vi "3d_display2.vi"() -> ()   [LabVIEW 2009]
doc: "This example demonstrates some fundamental concepts for the 3D picture control. Concepts covered include:\n\n-Object creation\n-Texturing\n-Object movement\n-Object hierarchy"
uses:
  <vilib>/Utility/miscctls.llb/LVRectTypeDef.ctl
  <vilib>/picture/3D Picture Control/NI_3D Picture Control.lvlib
  <vilib>/Analysis/NI_AALBase.lvlib
panel:
  out "Numeric 2":dbl
  out "Numeric":dbl
  in  "Set Start Time (s)":dbl
  in  "X":dbl
  in  "Z":dbl
  in  "Calibrate Z":bool
  in  "Calibrate Y":bool
  in  "Calibrate X":bool
  out "angle 2":dbl
  out "angle 1":dbl
  out "X mean acceleration":dbl format="%0.4f"
  out "Y mean acceleration":dbl format="%0.4f"
  out "X mean volts":dbl format="%0.4f"
  out "Y mean volts":dbl format="%0.4f"
  out "Z mean acceleration":dbl format="%0.4f"
  out "Z mean volts":dbl format="%0.4f"
  in  "z gain":dbl=5.0
  in  "z offset":dbl=1.25
  in  "y gain":dbl=5.0
  in  "y offset":dbl=1.25
  in  "x gain":dbl=5.0
  in  "x offset":dbl=1.25
  in  "Render Dest":enum16{"Scene Window", "Scene Display"}(ring)
  in  "Camera Controller":enum16{"None", "Spherical", "Flying"}(ring)=enum."Spherical"
  out "Scene Display":refnum<vi>(3d-picture)
  in  "stop":bool
  # "Select 'Render Dest'\nbefore running!"
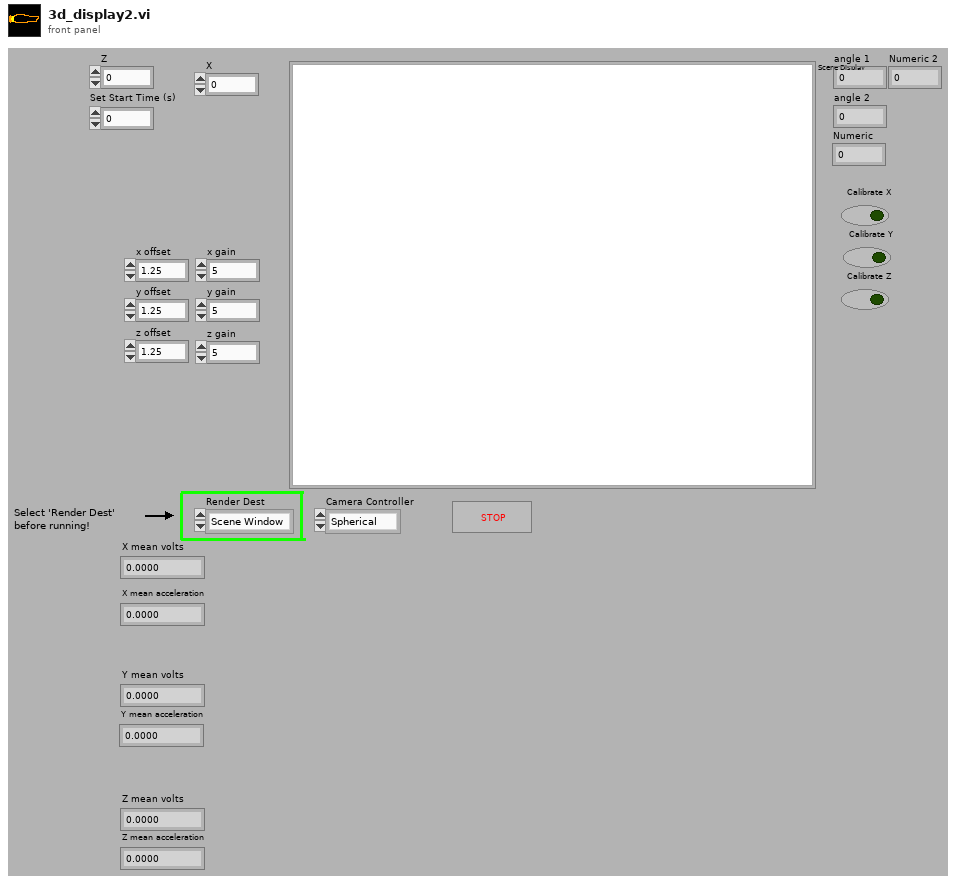
[diagram p1: front panel]
types:
  T1 = typedef "LVRectTypeDef.ctl" = cluster{"Left":i16, "Top":i16, "Right":i16, "Bottom":i16}
  T2 = enum16{"Open", "Minimized", "Maximized", "Hidden"}
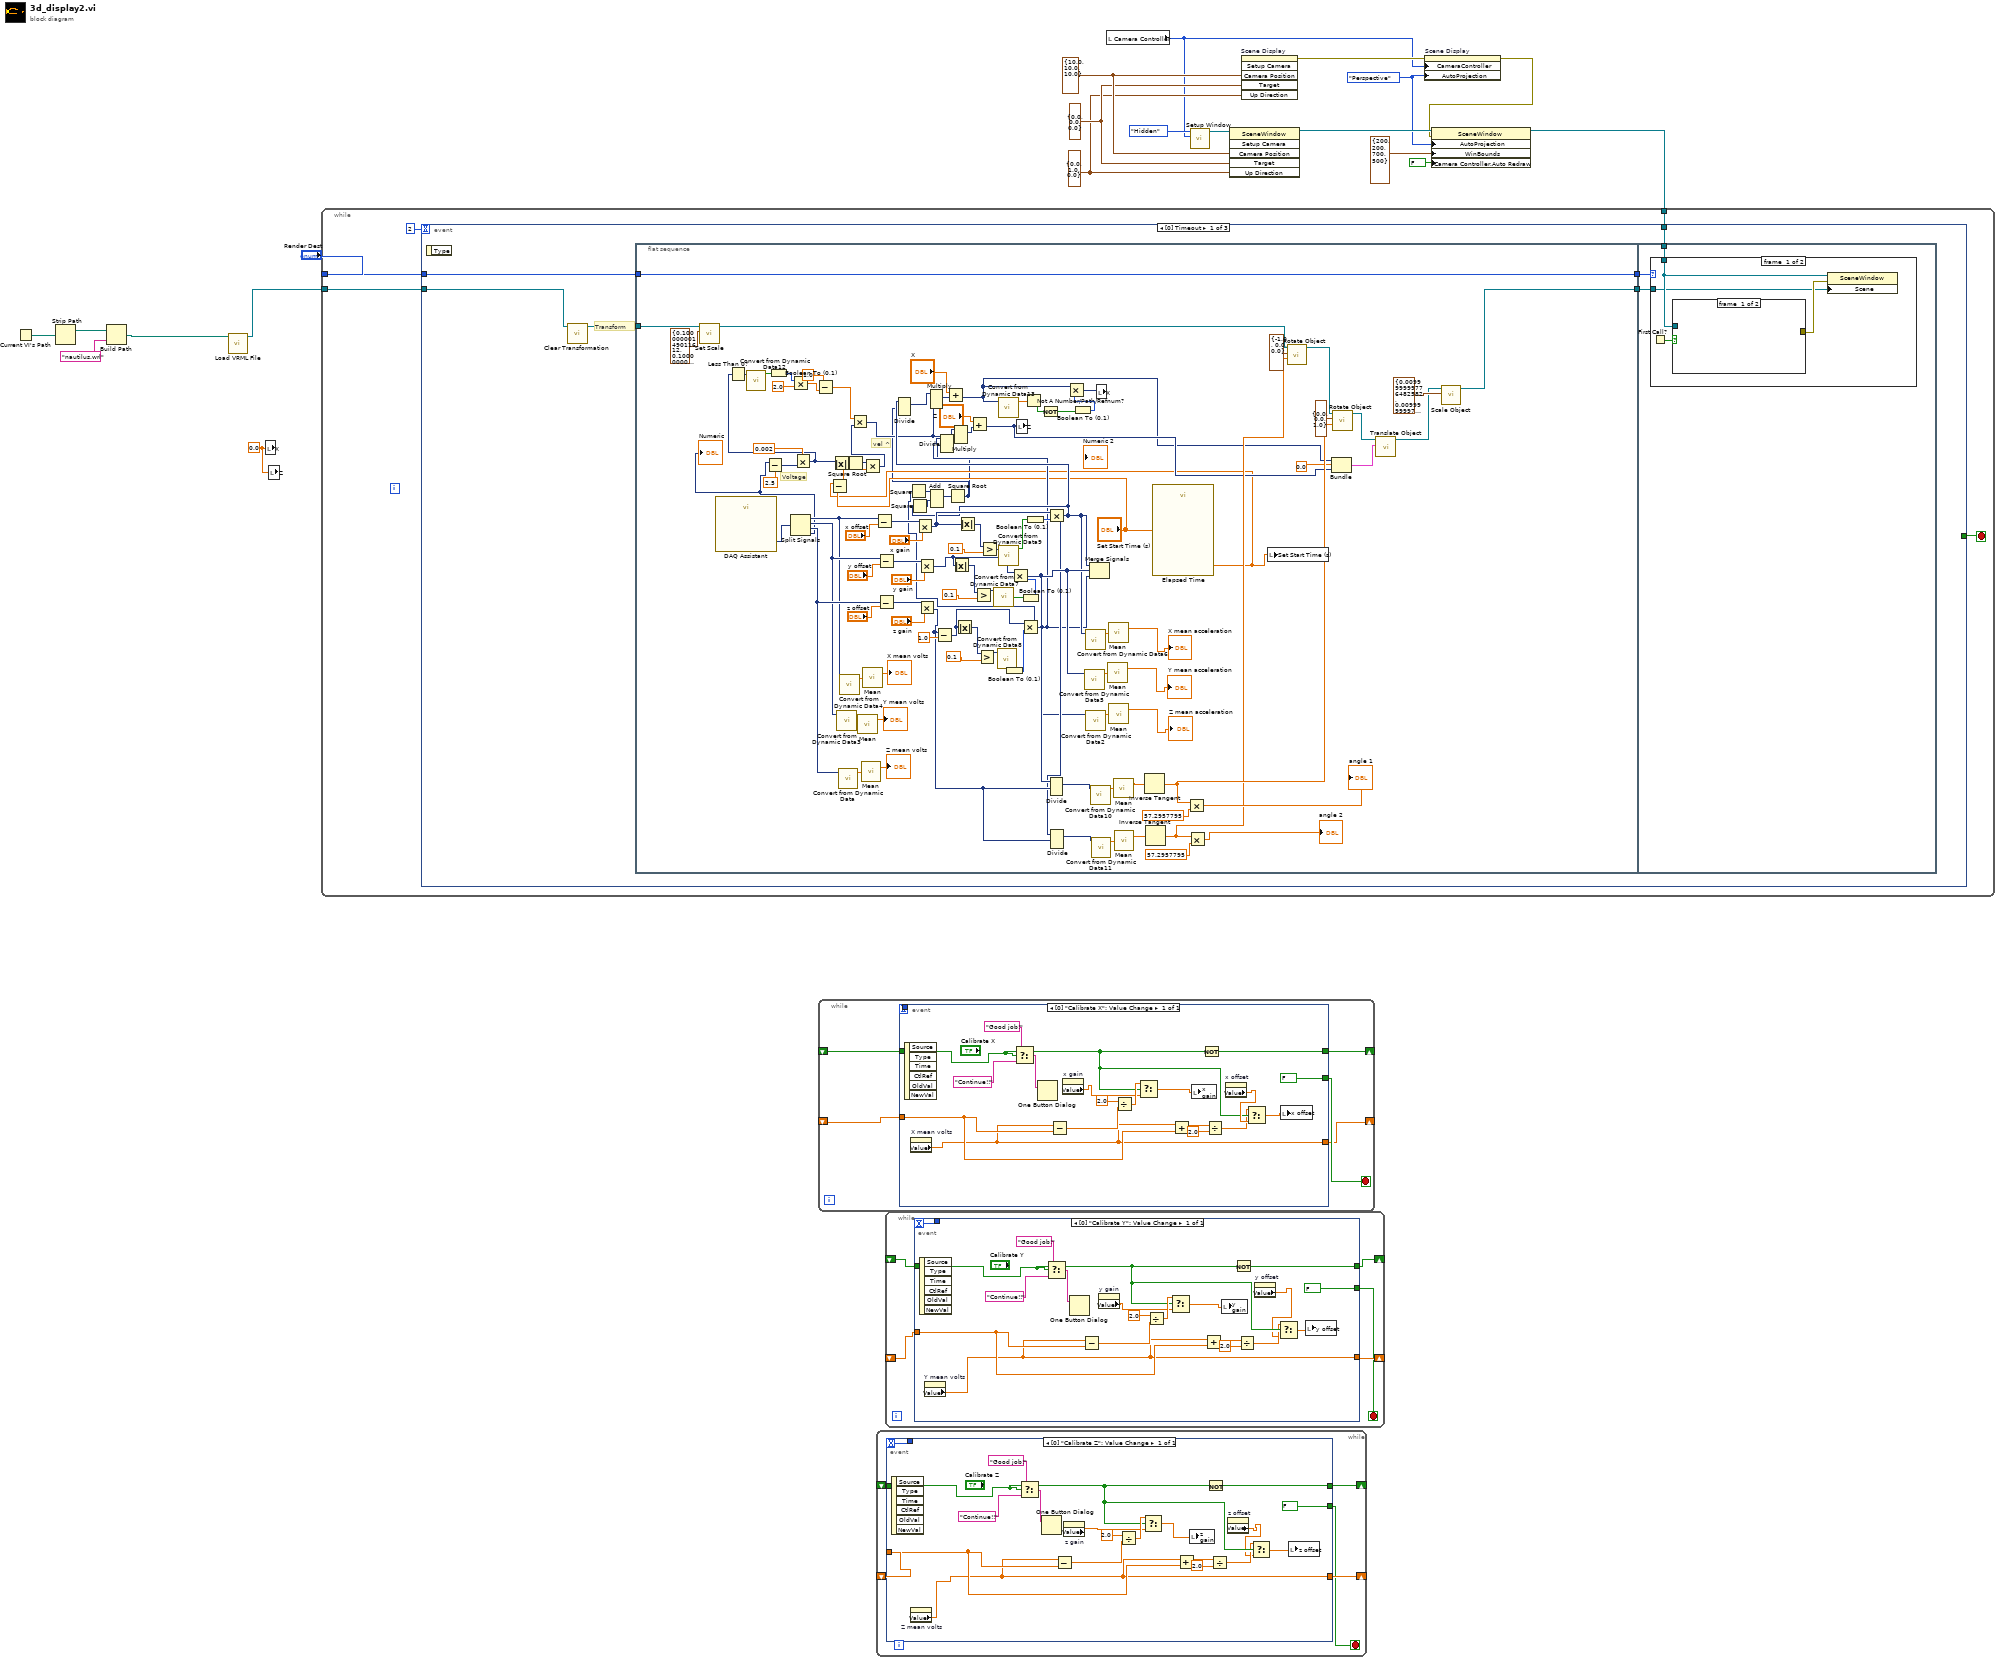
[diagram p0: block diagram]
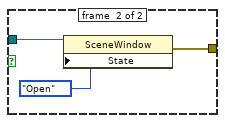
[diagram p2: hidden frame]
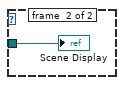
[diagram p3: hidden frame]
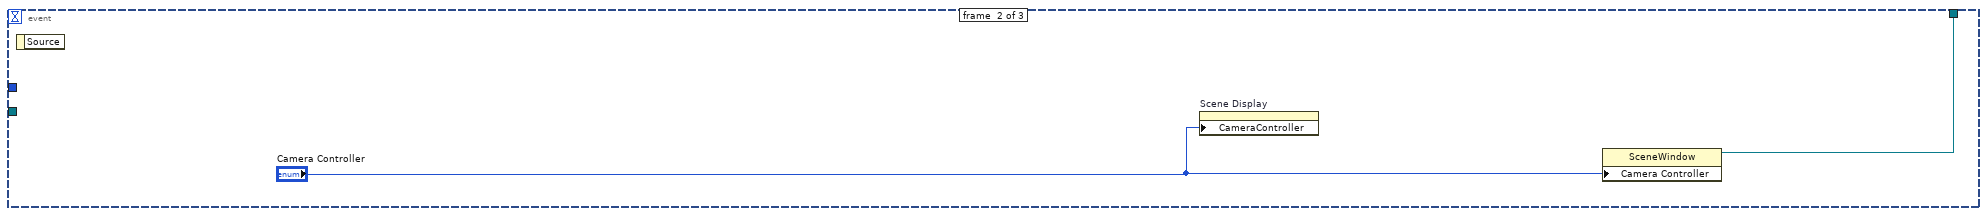
[diagram p4: hidden frame]
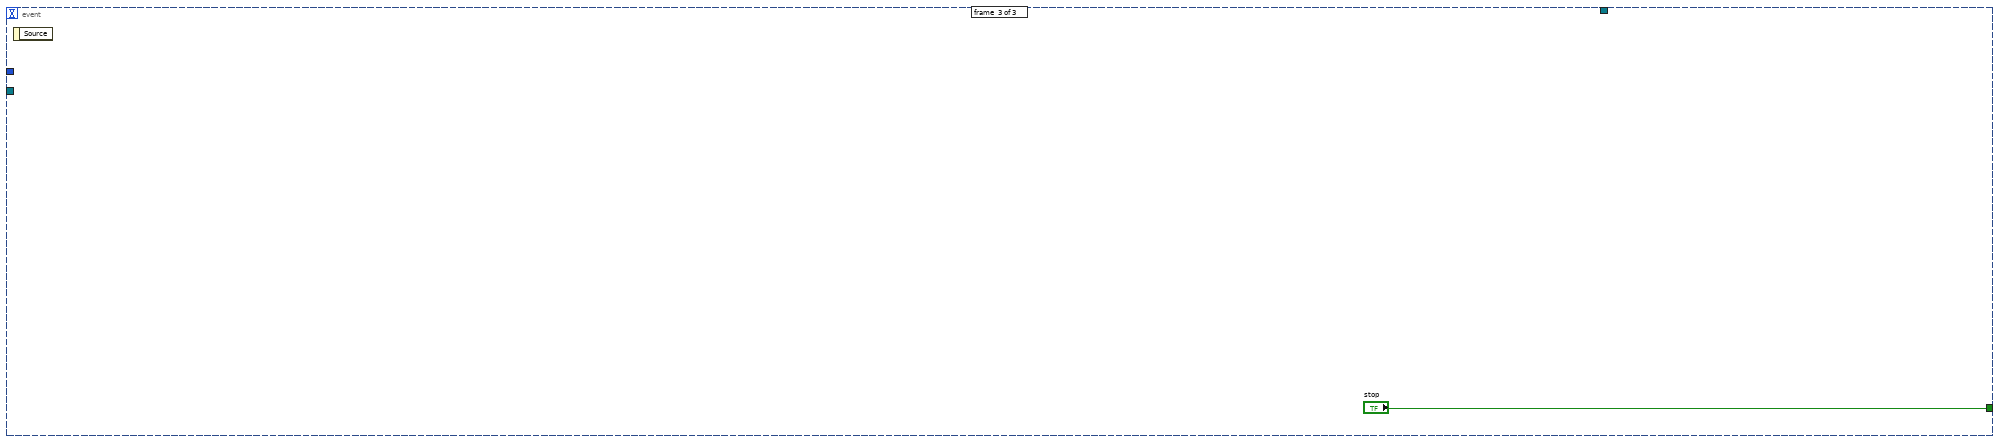
[diagram p5: hidden frame]
diagram:
  w1 = 0.0 ("X")
  w13 = enum16{"None", "Perspective", "Orthographic"}."Perspective" ("Auto Projection Mode")
  w16 = cluster{"X":sgl, "Y":sgl, "Z":sgl} {"X"=0.0, "Y"=1.0, "Z"=0.0} ("Up Direction")
  w17 = cluster{"X":sgl, "Y":sgl, "Z":sgl} {"X"=0.0, "Y"=0.0, "Z"=0.0} ("Target")
  w18 = cluster{"X":sgl, "Y":sgl, "Z":sgl} {"X"=10.0, "Y"=10.0, "Z"=10.0} ("Camera Position")
  n1 = Current VI's Path() -> (path=w5:path)
  n2 = Strip Path(path=w5) -> (stripped path=w6:path)  [unwired: 1 out]
  n3 = Build Path(base path=w6, name or relative path="nautilus.wrl") -> (appended path=w3:path)
  n4 = call <vilib>:"Load VRML File.vi"("Path"=w3) -> ("Scene:Read Scene File"=w2:refnum<vi>)  [unwired: 9 in, 1 out]
  n5 = local write "X"(w1) -> ()
  n6 = local write "Z"(w1) -> ()
  n7 = while {
    shift-right: [w23] -> _
    shift-left: _ -> [w24]
    shift-right: [w22] -> _
    shift-left: _ -> [w21]
    stop <- w25 stop-if-true
    n8 = event shown="[0] \"Calibrate X\": Value Change" {
      selector: _ -> [_]
      dyn-events: _ -> [_]
      timeout: _ -> [w44]
      tunnel: [w44] -> _
      tunnel: [FALSE ("Run")] -> w25
      tunnel: w24 -> [w31]
      tunnel: [w39] -> w23
      tunnel: [w26] -> w22
      tunnel: w21 -> [w30]
      event [0] "Calibrate X": Value Change {
        n9 = event-data() -> ()  [unwired: 1 in, 6 out]
        n10 = property on="X mean volts" class="DigNum (strict)"() -> ("Value"=w26:dbl)  [unwired: 2 in, 2 out]
        n11 = Select(t="Good job!" ("message"), s=w31, f="Continue!!" ("message")) -> (s? t:f=w43:string)
        n12 = One Button Dialog(message=w43) -> ()  [unwired: 1 in, 1 out]
        n13 = Subtract(x=w26, y=w30) -> (x-y=w37:dbl)
        n14 = property on="x gain" class="DigNum (strict)"() -> ("Value"=w35:dbl)  [unwired: 2 in, 2 out]
        n15 = Divide(x=2.0, y=w37) -> (x/y=w36:dbl)
        n16 = Select(t=w36, s=w31, f=w35) -> (s? t:f=w34:dbl)
        n17 = Add(x=w26, y=w30) -> (x+y=w28:dbl)
        n18 = local write "x gain"(w34) -> ()
        n19 = Not(x=w31) -> (.not. x?=w39:bool)
        n20 = Divide(x=w28, y=2.0) -> (x/y=w27:dbl)
        n21 = property on="x offset" class="DigNum (strict)"() -> ("Value"=w32:dbl)  [unwired: 2 in, 2 out]
        n22 = Select(t=w27, s=w31, f=w32) -> (s? t:f=w33:dbl)
        n23 = local write "x offset"(w33) -> ()
      }
    }
  }
  n24 = while {
    shift-right: [w47] -> _
    shift-left: _ -> [w46]
    shift-right: [w49] -> _
    shift-left: _ -> [w48]
    stop <- w45 stop-if-true
    n25 = event shown="[0] \"Calibrate Z\": Value Change" {
      selector: _ -> [_]
      dyn-events: _ -> [_]
      timeout: _ -> [w68]
      tunnel: [w68] -> _
      tunnel: w48 -> [w60]
      tunnel: [w64] -> w49
      tunnel: [w50] -> w47
      tunnel: w46 -> [w59]
      tunnel: [FALSE ("Run")] -> w45
      event [0] "Calibrate Z": Value Change {
        n26 = event-data() -> ()  [unwired: 1 in, 6 out]
        n27 = property on="Z mean volts" class="DigNum (strict)"() -> ("Value"=w50:dbl)  [unwired: 2 in, 2 out]
        n28 = Select(t="Good job!" ("message"), s=w60, f="Continue!!" ("message")) -> (s? t:f=w67:string)
        n29 = One Button Dialog(message=w67) -> ()  [unwired: 1 in, 1 out]
        n30 = Subtract(x=w50, y=w59) -> (x-y=w62:dbl)
        n31 = property on="z gain" class="DigNum (strict)"() -> ("Value"=w54:dbl)  [unwired: 2 in, 2 out]
        n32 = Divide(x=2.0, y=w62) -> (x/y=w61:dbl)
        n33 = Select(t=w61, s=w60, f=w54) -> (s? t:f=w52:dbl)
        n34 = Add(x=w50, y=w59) -> (x+y=w57:dbl)
        n35 = local write "z gain"(w52) -> ()
        n36 = Not(x=w60) -> (.not. x?=w64:bool)
        n37 = Divide(x=w57, y=2.0) -> (x/y=w56:dbl)
        n38 = property on="z offset" class="DigNum (strict)"() -> ("Value"=w53:dbl)  [unwired: 2 in, 2 out]
        n39 = Select(t=w56, s=w60, f=w53) -> (s? t:f=w55:dbl)
        n40 = local write "z offset"(w55) -> ()
      }
    }
  }
  n41 = while {
    shift-right: [w73] -> _
    shift-left: _ -> [w72]
    shift-right: [w70] -> _
    shift-left: _ -> [w71]
    stop <- w69 stop-if-true
    n42 = event shown="[0] \"Calibrate Y\": Value Change" {
      selector: _ -> [_]
      dyn-events: _ -> [_]
      timeout: _ -> [w92]
      tunnel: [w92] -> _
      tunnel: w72 -> [w84]
      tunnel: [w88] -> w73
      tunnel: [w74] -> w70
      tunnel: w71 -> [w83]
      tunnel: [FALSE ("Run")] -> w69
      event [0] "Calibrate Y": Value Change {
        n43 = event-data() -> ()  [unwired: 1 in, 6 out]
        n44 = property on="Y mean volts" class="DigNum (strict)"() -> ("Value"=w74:dbl)  [unwired: 2 in, 2 out]
        n45 = Select(t="Good job!" ("message"), s=w84, f="Continue!!" ("message")) -> (s? t:f=w91:string)
        n46 = One Button Dialog(message=w91) -> ()  [unwired: 1 in, 1 out]
        n47 = Subtract(x=w74, y=w83) -> (x-y=w86:dbl)
        n48 = property on="y gain" class="DigNum (strict)"() -> ("Value"=w79:dbl)  [unwired: 2 in, 2 out]
        n49 = Divide(x=2.0, y=w86) -> (x/y=w85:dbl)
        n50 = Select(t=w85, s=w84, f=w79) -> (s? t:f=w78:dbl)
        n51 = Add(x=w74, y=w83) -> (x+y=w81:dbl)
        n52 = local write "y gain"(w78) -> ()
        n53 = Not(x=w84) -> (.not. x?=w88:bool)
        n54 = Divide(x=w81, y=2.0) -> (x/y=w80:dbl)
        n55 = property on="y offset" class="DigNum (strict)"() -> ("Value"=w77:dbl)  [unwired: 2 in, 2 out]
        n56 = Select(t=w80, s=w84, f=w77) -> (s? t:f=w76:dbl)
        n57 = local write "y offset"(w76) -> ()
      }
    }
  }
  n58 = local read "Camera Controller"() -> (w10:enum16{"None", "Spherical", "Flying"})
  n59 = call <vilib>:"Setup Window.vi"("Camera Controller"=w10, "Window State"=T2."Hidden") -> ("New Window Refnum"=w12:refnum<vi>)  [unwired: 1 in, 8 out]
  n60 = invoke class="SceneWindow" method="Setup Camera"(reference=w12, "Camera Position"=w18, "Target"=w17, "Up Direction"=w16) -> (reference out=w20:refnum<vi>)  [unwired: 2 in, 5 out]
  n61 = invoke on="Scene Display" class="SceneGraphDisp (strict)" method="Setup Camera"("Camera Position"=w18, "Target"=w17, "Up Direction"=w16) -> (error out=w15:errorcluster)  [unwired: 3 in, 5 out]
  n62 = property on="Scene Display" class="SceneGraphDisp (strict)"(error in=w15, "CameraController"=w10, "AutoProjection"=w13) -> (error out=w14:errorcluster)  [unwired: 1 in, 1 out]
  n63 = property class="SceneWindow"(reference=w20, error in=w14, "AutoProjection"=w13, "WinBounds"=T1 {"Left"=200, "Top"=200, "Right"=700, "Bottom"=500} ("Window Bounds"), "Camera Controller.Auto Redraw"=FALSE ("Camera Controller:Auto Redraw")) -> (reference out=w8:refnum<vi>)  [unwired: 1 out]
  n64 = while {
    tunnel: w8 -> [w97]
    tunnel: w2 -> [w96]
    tunnel: "Render Dest" -> [w93]
    stop <- w94 stop-if-true
    n65 = event shown="[0] Timeout" {
      selector: _ -> [_ _ _]
      dyn-events: _ -> [_ _ _]
      timeout: 2 -> [_ _ _]
      tunnel: w97 -> [w103 w225 _]
      tunnel: w96 -> [w99 _ _]
      tunnel: [_ _ "stop"] -> w94
      tunnel: w93 -> [w100 _ _]
      event #0 {
        # "Transform"
        n66 = event-data() -> ()  [unwired: 2 out]
        n67 = call <vilib>:"Clear Transformation.vi"("Object Refnum In"=w99) -> ("Object Refnum Out"=w102:refnum<vi>)  [unwired: 1 in, 9 out]
        n68 = flat-sequence {
          tunnel: w102 -> [w113]
          tunnel: [w212] -> w101
          tunnel: w100 -> [w212]
          tunnel: [w209] -> w98
          tunnel: w103 -> [w215]
          tunnel: w101 -> [w214]
          tunnel: w98 -> [w213]
          frame #0 {
            # "vel ^"
            # "Voltage"
            n69 = call <vilib>:"Set Scale.vi"("Scale"=cluster{"X":sgl, "Y":sgl, "Z":sgl} {"X"=0.1, "Y"=0.1, "Z"=0.1}, "Scene Object"=w113) -> ("Scaled Object"=w112:refnum<vi>)  [unwired: 8 in, 1 out]
            n70 = call "DAQ Assistant"() -> ("data"=w152:dynamicdata)  [unwired: 17 in, 2 out]
            n71 = Split Signals(w152) -> (w192:dynamicdata, w194:dynamicdata, w197:dynamicdata, w118:dynamicdata)  [unwired: 4 in]
            "Numeric" <- w118
            n72 = Subtract(x=w118, y=2.5) -> (x-y=w147:dynamicdata)
            n73 = Multiply(x=0.002, y=w147) -> (x*y=w117:dynamicdata)
            n74 = Less Than 0?(x=w117) -> (x < 0?=w126:dynamicdata)
            n75 = call "Convert from Dynamic Data12"("Dynamic Data Type"=w126) -> ("Scalar"=w125:bool)  [unwired: 3 in]
            n76 = Boolean To (0,1)(Boolean=w125) -> (0, 1=w123:i16)
            n77 = Multiply(x=w123, y=2.0) -> (x*y=w121:dbl)
            n78 = Subtract(x=1.0 ("y"), y=w121) -> (x-y=w116:dbl)
            n79 = Absolute Value(x=w117) -> (abs(x)=w120:dynamicdata)
            n80 = call "Convert from Dynamic Data3"("Dynamic Data Type"=w194) -> ("Array"=w193:dbl[])  [unwired: 3 in]
            n81 = call "Convert from Dynamic Data"("Dynamic Data Type"=w197) -> ("Array"=w199:dbl[])  [unwired: 3 in]
            n82 = call "Convert from Dynamic Data4"("Dynamic Data Type"=w192) -> ("Array"=w191:dbl[])  [unwired: 3 in]
            n83 = Square Root(x=w120) -> (sqrt(x)=w119:dynamicdata)
            n84 = call <vilib>:"Mean.vi"("X"=w193) -> ("mean"=→"Y mean volts":dbl)  [unwired: 1 out]
            n85 = call <vilib>:"Mean.vi"("X"=w199) -> ("mean"=→"Z mean volts":dbl)  [unwired: 1 out]
            n86 = call <vilib>:"Mean.vi"("X"=w191) -> ("mean"=→"X mean volts":dbl)  [unwired: 1 out]
            n87 = Subtract(x=w192, y="x offset") -> (x-y=w208:dynamicdata)
            n88 = Subtract(x=w194, y="y offset") -> (x-y=w204:dynamicdata)
            n89 = Subtract(x=w197, y="z offset") -> (x-y=w186:dynamicdata)
            n90 = Multiply(x=w208, y="x gain") -> (x*y=w167:dynamicdata)
            n91 = Multiply(x=w204, y="y gain") -> (x*y=w185:dynamicdata)
            n92 = Multiply(x=w186, y="z gain") -> (x*y=w156:dynamicdata)
            n93 = Subtract(x=w156, y=1.0) -> (x-y=w173:dynamicdata)
            n94 = Absolute Value(x=w185) -> (abs(x)=w184:dynamicdata)
            n95 = Absolute Value(x=w173) -> (abs(x)=w179:dynamicdata)
            n96 = Absolute Value(x=w167) -> (abs(x)=w172:dynamicdata)
            n97 = Greater?(x=w184, y=0.1) -> (0:w181:dynamicdata)
            n98 = Greater?(x=w179, y=0.1) -> (0:w177:dynamicdata)
            n99 = Greater?(x=w172, y=0.1) -> (0:w169:dynamicdata)
            n100 = call "Convert from Dynamic Data7"("Dynamic Data Type"=w181) -> ("Scalar"=w180:bool)  [unwired: 3 in]
            n101 = call "Convert from Dynamic Data8"("Dynamic Data Type"=w177) -> ("Scalar"=w176:bool)  [unwired: 3 in]
            n102 = call "Convert from Dynamic Data9"("Dynamic Data Type"=w169) -> ("Scalar"=w168:bool)  [unwired: 3 in]
            n103 = Boolean To (0,1)(Boolean=w176) -> (0, 1=w175:i16)
            n104 = Boolean To (0,1)(Boolean=w180) -> (0, 1=w182:i16)
            n105 = Multiply(x=w185, y=w182) -> (x*y=w162:dynamicdata)
            n106 = Multiply(x=w173, y=w175) -> (x*y=w136:dynamicdata)
            n107 = Square(x=w136) -> (x^2=w142:dynamicdata)
            n108 = Boolean To (0,1)(Boolean=w168) -> (0, 1=w170:i16)
            n109 = Divide(1:w156, 2:w162) -> (0:w164:dynamicdata)  [unwired: 1 in, 1 out]
            n110 = Multiply(x=w167, y=w170) -> (x*y=w137:dynamicdata)
            n111 = Square(x=w137) -> (x^2=w143:dynamicdata)
            n112 = Add(1:w143, 2:w142) -> (0:w141:dynamicdata)  [unwired: 1 in, 1 out]
            n113 = Square Root(x=w141) -> (sqrt(x)=w110:dynamicdata)
            n114 = Divide(1:w110, 2:w137) -> (0:w139:dynamicdata)  [unwired: 1 in, 1 out]
            n115 = Divide(1:w110, 2:w136) -> (0:w138:dynamicdata)  [unwired: 1 in, 1 out]
            n116 = Divide(1:w156, 2:w137) -> (0:w158:dynamicdata)  [unwired: 1 in, 1 out]
            n117 = call "Convert from Dynamic Data5"("Dynamic Data Type"=w162) -> ("Array"=w188:dbl[])  [unwired: 3 in]
            n118 = call "Convert from Dynamic Data6"("Dynamic Data Type"=w137) -> ("Array"=w187:dbl[])  [unwired: 3 in]
            n119 = call "Convert from Dynamic Data2"("Dynamic Data Type"=w136) -> ("Array"=w198:dbl[])  [unwired: 3 in]
            n120 = Merge Signals(w137, w162, w136) -> ()  [unwired: 1 out]
            n121 = call "Convert from Dynamic Data10"("Dynamic Data Type"=w164) -> ("Array"=w166:dbl[])  [unwired: 3 in]
            n122 = call "Convert from Dynamic Data11"("Dynamic Data Type"=w158) -> ("Array"=w160:dbl[])  [unwired: 3 in]
            n123 = call <vilib>:"Mean.vi"("X"=w188) -> ("mean"=→"Y mean acceleration":dbl)  [unwired: 1 out]
            n124 = call <vilib>:"Mean.vi"("X"=w187) -> ("mean"=→"X mean acceleration":dbl)  [unwired: 1 out]
            n125 = call <vilib>:"Mean.vi"("X"=w198) -> ("mean"=→"Z mean acceleration":dbl)  [unwired: 1 out]
            n126 = call <vilib>:"Mean.vi"("X"=w166) -> ("mean"=w165:dbl)  [unwired: 1 out]
            n127 = call <vilib>:"Mean.vi"("X"=w160) -> ("mean"=w159:dbl)  [unwired: 1 out]
            n128 = Inverse Tangent(1:w165) -> (0:w151:dbl)
            n129 = Inverse Tangent(1:w159) -> (0:w150:dbl)
            n130 = call "Elapsed Time"("Set Start Time (s)"="Set Start Time (s)") -> ("Present (s)"=w128:dbl)  [unwired: 11 in, 7 out]
            n131 = Subtract(x=w128, y="Set Start Time (s)") -> (x-y=w127:dbl)
            n132 = Multiply(x=w119, y=w127) -> (x*y=w115:dynamicdata)
            n133 = Multiply(x=w116, y=w115) -> (x*y=w114:dynamicdata)
            n134 = Multiply(1:w114, 2:w139) -> (0:w140:dynamicdata)  [unwired: 1 in, 1 out]
            n135 = Add(x="X", y=w140) -> (x+y=w108:dynamicdata)
            n136 = Multiply(1:w114, 2:w138) -> (0:w135:dynamicdata)  [unwired: 1 in, 1 out]
            n137 = Add(x="Z", y=w135) -> (x+y=w131:dynamicdata)
            n138 = call "Convert from Dynamic Data13"("Dynamic Data Type"=w108) -> ("Scalar"=w109:dbl)  [unwired: 3 in]
            n139 = local write "Z"(w131) -> ()
            n140 = Not A Number/Path/Refnum?(number/path/refnum=w109) -> (NaN/Path/Refnum?=w105:bool)
            n141 = Not(x=w105) -> (.not. x?=w104:bool)
            n142 = Boolean To (0,1)(Boolean=w104) -> (0, 1=w107:i16)
            n143 = Multiply(x=w108, y=w107) -> (x*y=w106:dynamicdata)
            n144 = local write "X"(w106) -> ()
            n145 = Multiply(x=w151, y=57.2957795) -> (x*y=→"angle 1":dbl)
            n146 = Multiply(x=w150, y=57.2957795) -> (x*y=→"angle 2":dbl)
            n147 = local write "Set Start Time (s)"(w128) -> ()
            n148 = call <vilib>:"Rotate Object.vi"("Angle"=w150, "Axis"=cluster{"X":sgl, "Y":sgl, "Z":sgl} {"X"=-1.0, "Y"=0.0, "Z"=0.0}, "Scene.Object In"=w112) -> ("Scene.Object Out"=w154:refnum<vi>)  [unwired: 7 in, 1 out]
            n149 = Bundle(w108, "element"=0.0, w131) -> (w130:cluster{dynamicdata, "element":dbl, dynamicdata})  [unwired: 1 in]
            n150 = call <vilib>:"Rotate Object.vi"("Angle"=w151, "Axis"=cluster{"X":sgl, "Y":sgl, "Z":sgl} {"X"=0.0, "Y"=0.0, "Z"=1.0}, "Scene.Object In"=w154) -> ("Scene.Object Out"=w134:refnum<vi>)  [unwired: 7 in, 1 out]
            n151 = call <vilib>:"Translate Object.vi"("Translation"=w130, "Scene.Object In"=w134) -> ("Scene.Object Out"=w133:refnum<vi>)  [unwired: 8 in, 1 out]
            n152 = call <vilib>:"Scale Object.vi"("Scale"=cluster{"X":sgl, "Y":sgl, "Z":sgl} {"X"=0.01, "Y"=0.01, "Z"=0.01}, "Scene.Object In"=w133) -> ("Scene.Object Out"=w209:refnum<vi>)  [unwired: 8 in, 1 out]
          }
          frame #1 {
            n153 = case shown="\"Scene Window\", Default" w214 {
              tunnel: w215 -> [w219 _]
              tunnel: w213 -> [w216 w223]
              frame #0 {
                n154 = First Call?() -> (First Call?: T/F=w217:bool)
                n155 = case shown="True" w217 {
                  tunnel: w219 -> [_ w222]
                  tunnel: [_ w221] -> w218
                  frame #0 {
                  }
                  frame #1 {
                    n156 = property class="SceneWindow"(reference=w222, "State"=T2."Open" ("Window State")) -> (error out=w221:errorcluster)  [unwired: 1 in, 1 out]
                  }
                }
                n157 = property class="SceneWindow"(reference=w219, error in=w218, "Scene"=w216) -> ()  [unwired: 2 out]
              }
              frame #1 {
                "Scene Display" <- w223
              }
            }
          }
        }
      }
      event #1 {
        n158 = event-data() -> ()  [unwired: 2 out]
        n159 = property on="Scene Display" class="SceneGraphDisp (strict)"("CameraController"="Camera Controller") -> ()  [unwired: 2 in, 2 out]
        n160 = property class="SceneWindow"(reference=w225, "Camera Controller"="Camera Controller") -> ()  [unwired: 1 in, 2 out]
      }
      event #2 {
        n161 = event-data() -> ()  [unwired: 2 out]
      }
    }
  }
